vi "testCaseStructure.vi"() -> ()   [LabVIEW 2014]
uses:
  mainMachine.ctl
  testMachine.ctl
panel:
  out "data":dynamicdata(graph)
  out "ledEnsaio":bool caption="Ensaio"
  out "ledExit":bool caption="Exit State"
  out "ledBrake":bool caption="Brake State"
  out "ledMotor":bool caption="Motor State"
  out "ledInit2":bool caption="Init State"
  out "ledFinish":bool caption="Finish State"
  out "testMachine":T1=enum."exit"
  out "mainMachine":T2
  out "ledStop":bool caption="Block State"
  out "ledRunning":bool caption="Running State"
  out "ledReady":bool caption="Ready State"
  in  "buttonStop":bool
  in  "buttonStart":bool
  out "ledInit":bool caption="Init State"
  in  "stop":bool
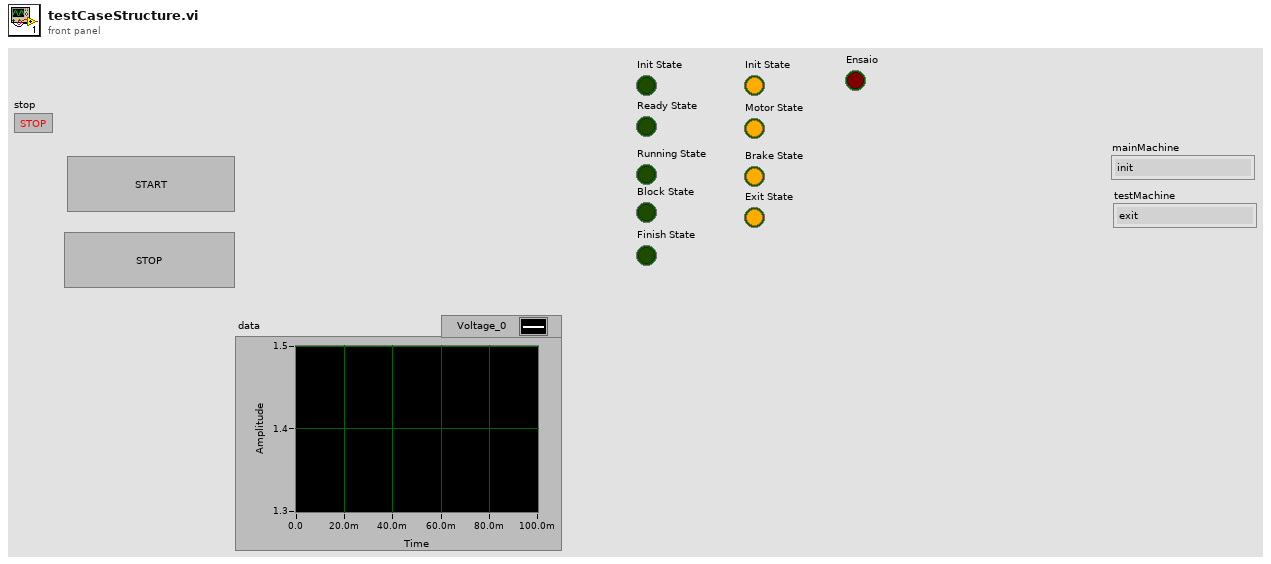
[diagram p1: front panel]
types:
  T1 = typedef "testMachine.ctl" = enum16{"init", "motor", "motor acquire", "brake acquire", "brake", "finish", "exit"}
  T2 = typedef "mainMachine.ctl" = enum16{"init", "ready", "running", "blocked", "finish"}
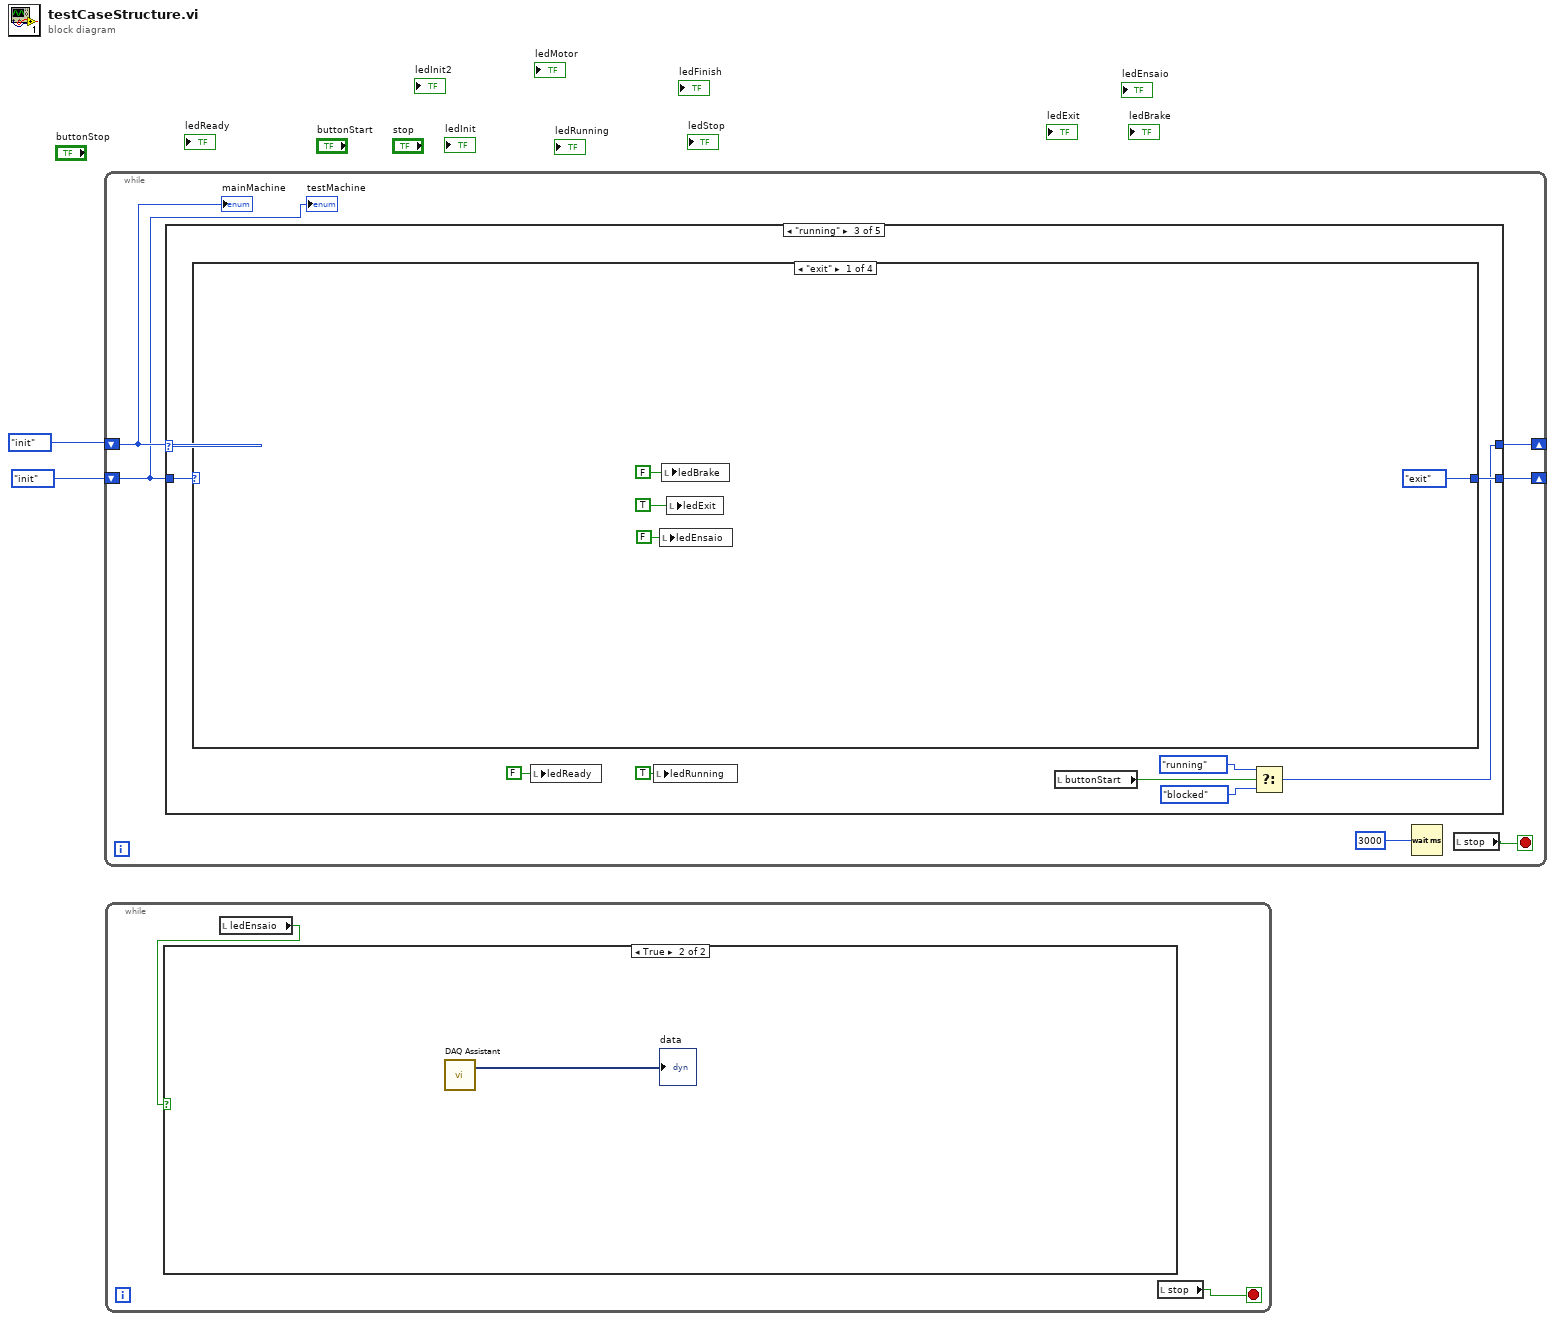
[diagram p0: block diagram]
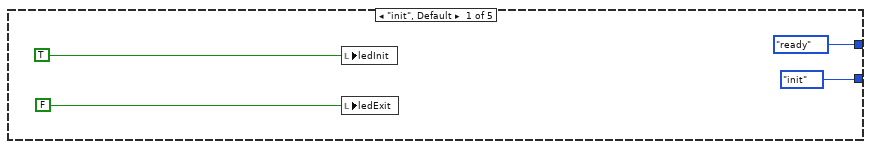
[diagram p3: hidden frame]
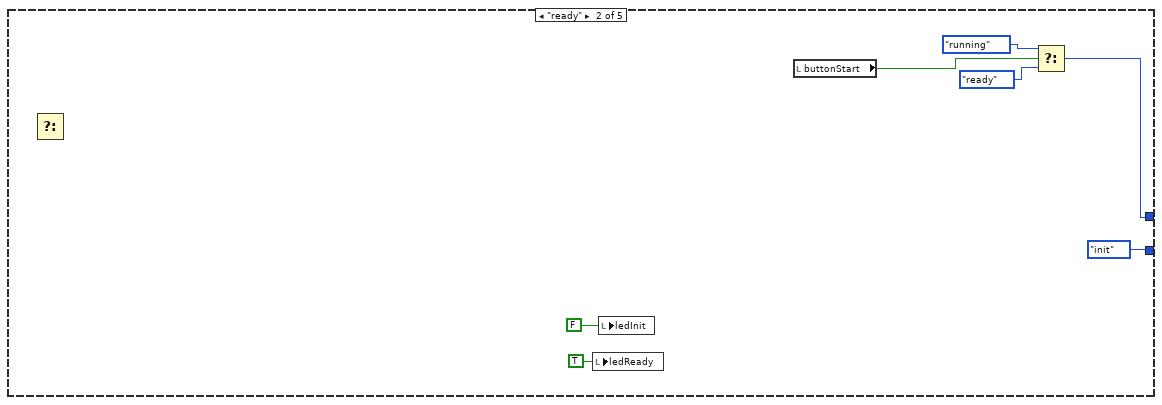
[diagram p4: hidden frame]
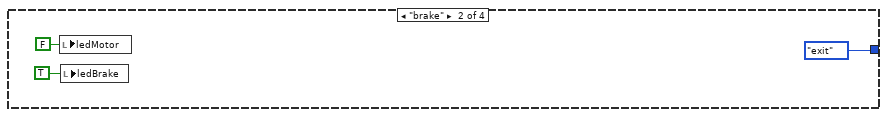
[diagram p5: hidden frame]
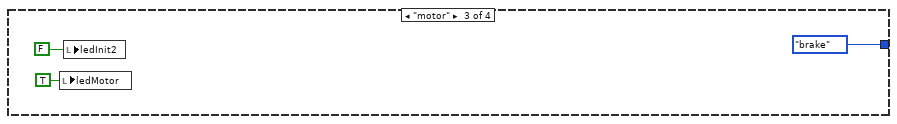
[diagram p6: hidden frame]
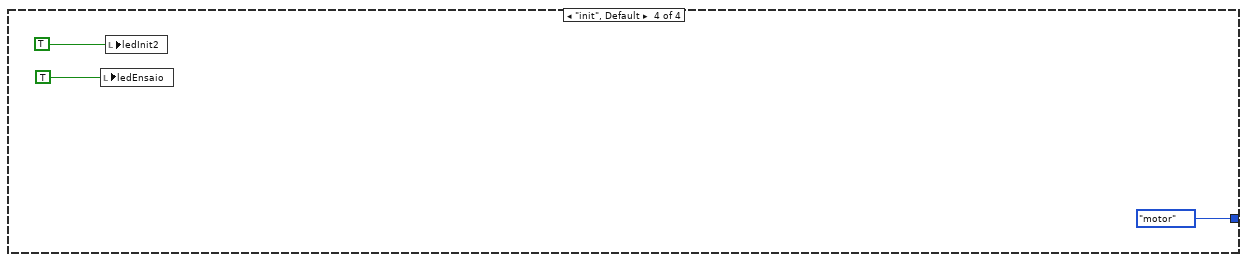
[diagram p7: hidden frame]
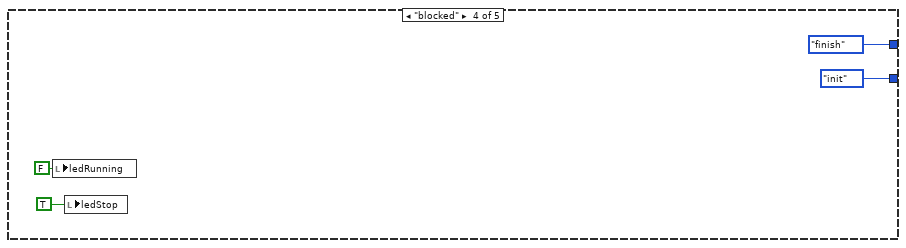
[diagram p8: hidden frame]
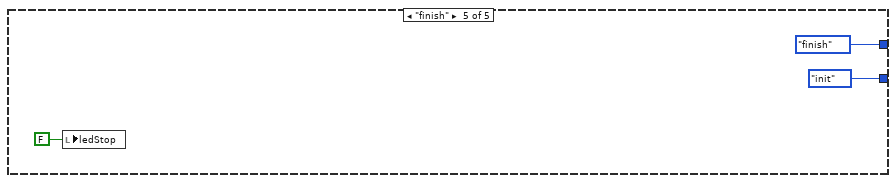
[diagram p9: hidden frame]
diagram:
  n1 = while {
    shift-right: [w5] -> _
    shift-left: mainMachine."init" ("mainMachine") -> [w6]
    shift-right: [w3] -> _
    shift-left: testMachine."init" ("testMachine") -> [w4]
    stop <- w8 stop-if-true
    n2 = case shown="\"running\"" w6 {
      tunnel: [mainMachine."ready" ("mainMachine") w17 w20 mainMachine."finish" ("mainMachine") mainMachine."finish" ("mainMachine")] -> w5
      tunnel: w4 -> [_ _ w27 _ _]
      tunnel: [testMachine."init" ("testMachine") testMachine."init" ("testMachine") w24 testMachine."init" ("testMachine") testMachine."init" ("testMachine")] -> w3
      frame "init", Default {
        n3 = local write "ledInit"(TRUE ("ledReady")) -> ()
        n4 = local write "ledExit"(FALSE ("ledReady")) -> ()
      }
      frame "ready" {
        n5 = Select() -> ()  [unwired: 3 in, 1 out]
        n6 = local write "ledReady"(TRUE ("ledReady")) -> ()
        n7 = local write "ledInit"(FALSE ("ledReady")) -> ()
        n8 = local read "buttonStart"() -> (w14:bool)
        n9 = Select(t=mainMachine."running" ("mainMachine"), s=w14, f=mainMachine."ready" ("mainMachine")) -> (s? t:f=w17:T2)
      }
      frame "running" {
        n10 = case shown="\"exit\"" w27 {
          tunnel: [testMachine."exit" ("testMachine") testMachine."exit" ("testMachine") testMachine."brake" ("testMachine") testMachine."motor" ("testMachine")] -> w24
          frame "exit" {
            n11 = local write "ledEnsaio"(FALSE ("ledReady")) -> ()
            n12 = local write "ledBrake"(FALSE ("ledReady")) -> ()
            n13 = local write "ledExit"(TRUE ("ledReady")) -> ()
          }
          frame "brake" {
            n14 = local write "ledMotor"(FALSE ("ledReady")) -> ()
            n15 = local write "ledBrake"(TRUE ("ledReady")) -> ()
          }
          frame "motor" {
            n16 = local write "ledMotor"(TRUE ("ledReady")) -> ()
            n17 = local write "ledInit2"(FALSE ("ledReady")) -> ()
          }
          frame "init", Default {
            n18 = local write "ledEnsaio"(TRUE ("ledReady")) -> ()
            n19 = local write "ledInit2"(TRUE ("ledReady")) -> ()
          }
        }
        n20 = local write "ledReady"(FALSE ("ledReady")) -> ()
        n21 = local write "ledRunning"(TRUE ("ledReady")) -> ()
        n22 = local read "buttonStart"() -> (w23:bool)
        n23 = Select(t=mainMachine."running" ("mainMachine"), s=w23, f=mainMachine."blocked" ("mainMachine")) -> (s? t:f=w20:T2)
      }
      frame "blocked" {
        n24 = local write "ledRunning"(FALSE ("ledReady")) -> ()
        n25 = local write "ledStop"(TRUE ("ledReady")) -> ()
      }
      frame "finish" {
        n26 = local write "ledStop"(FALSE ("ledReady")) -> ()
      }
    }
    n27 = Wait (ms)(milliseconds to wait=u32 3000) -> ()  [unwired: 1 out]
    n28 = local read "stop"() -> (w8:bool)
    "mainMachine" <- w6
    "testMachine" <- w4
  }
  n29 = while {
    stop <- w48 stop-if-true
    n30 = local read "ledEnsaio"() -> (w49:bool)
    n31 = case shown="True" w49 {
      frame False {
      }
      frame True {
        n32 = call "DAQ Assistant"() -> ("data"=→"data":dynamicdata)  [unwired: 16 in, 3 out]
      }
    }
    n33 = local read "stop"() -> (w48:bool)
  }
